vi "4155C Initialise.vi"(0 "VISA resource name in":refnum<visa-resource-name>, 1 "Reset":bool, 2 "Type of reset":u16(ring) items=["Reset All", "Partial reset"], 3 "error in (no error)":errorcluster, 4 "VISA Timeout Value":u32=10000) -> (5 "VISA Resource Name out":refnum<visa-resource-name>, 6 "error out":errorcluster)   [LabVIEW 2016]
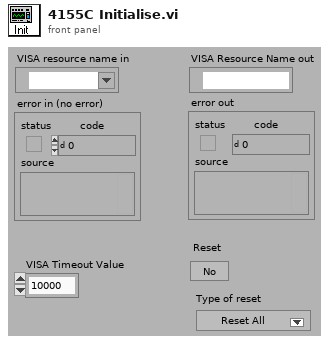
[diagram p1: front panel]
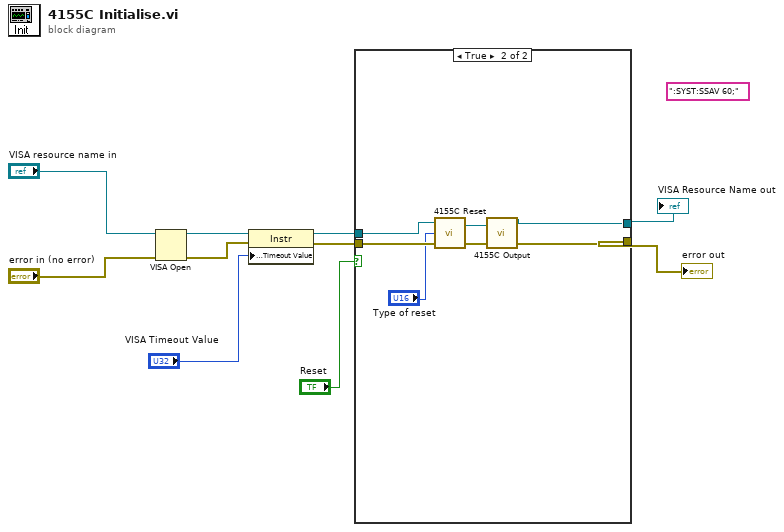
[diagram p0: block diagram]
diagram:
  (unwired) ":SYST:SSAV 60;" ("write buffer (\"\")")
  n1 = VISA Open(error in (no error)="error in (no error)", VISA resource name="VISA resource name in") -> (VISA resource name=w8:refnum<visa-resource-name>, error out=w7:errorcluster)  [unwired: 3 in]
  n2 = property class="Instr"(reference=w8, error in=w7, "General Settings:Timeout Value"="VISA Timeout Value") -> (reference out=w4:refnum<visa-resource-name>, error out=w3:errorcluster)
  n3 = case shown="True" "Reset" {
    tunnel: w4 -> [w12 w19]
    tunnel: w3 -> [w11 w18]
    tunnel: [w12 w13] -> w2
    tunnel: [w11 w14] -> w1
    frame False {
    }
    frame True {
      n4 = call "4155C Reset.vi"("error in (no error)"=w18, "Type of reset"="Type of reset", "VISA session"=w19) -> ("error out"=w15:errorcluster, "dup VISA resource name"=w16:refnum<visa-resource-name>)
      n5 = call "4155C Output.vi"("VISA resource name in"=w16, "error in (no error)"=w15) -> ("VISA Resource Name out"=w13:refnum<visa-resource-name>, "error out"=w14:errorcluster)  [unwired: 18 in, 6 out]
    }
  }
  "VISA Resource Name out" <- w2
  "error out" <- w1
